vi "calc_group_delay.vi"(8 "frequency+1":dbl, 9 "frequency":dbl, 10 "phase+1":dbl, 11 "phase":dbl) -> (3 "group_delay":dbl)   [LabVIEW 2025]
uses:
  <vilib>/Analysis/NI_AALPro.lvlib
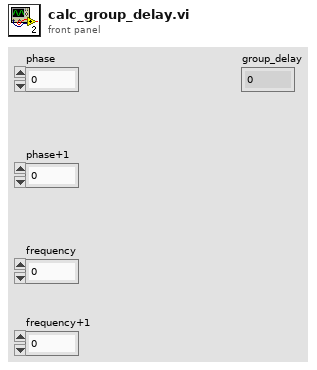
[diagram p1: front panel]
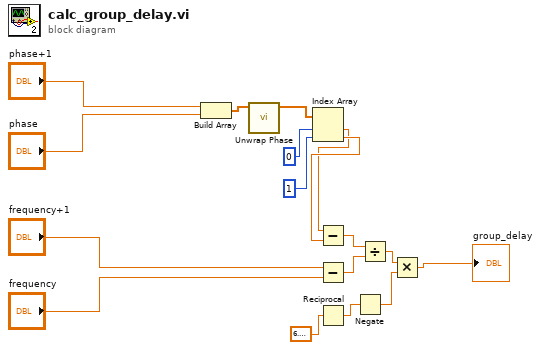
[diagram p0: block diagram]
diagram:
  n1 = Build Array("phase+1", "phase") -> (w11:dbl[])
  n2 = call <vilib>:"Unwrap Phase.vi"("Phase"=w11) -> ("Unwrapped Phase"=w12:dbl[])  [unwired: 9 in, 1 out]
  n3 = Index Array(array=w12, index #1=0 ("index"), index #2=1 ("index")) -> (element #1=w16:dbl, element #2=w17:dbl)
  n4 = Subtract(x=w16, y=w17) -> (x-y=w5:dbl)
  n5 = Subtract(x="frequency+1", y="frequency") -> (x-y=w6:dbl)
  n6 = Reciprocal(x=6.283185307179586) -> (1/x=w7:dbl)
  n7 = Negate(x=w7) -> (-x=w8:dbl)
  n8 = Divide(x=w5, y=w6) -> (x/y=w4:dbl)
  n9 = Multiply(x=w4, y=w8) -> (x*y=→"group_delay":dbl)
